vi "IDE_msg_Example.vi"() -> ()   [LabVIEW 2020]
uses:
  Subs/ColorText/Code.xctl
  Subs/Console XCtrl/Console_Xctrl.xctl
  Subs/Server XCtrl/Server.xctl
panel:
  in  "Clean":bool
  in  "PC Save":bool
  in  "PC path":path
  in  "Files":bool
  in  "Server":bool
  in  "Help":bool
  in  "Server":path(xcontrol)=path "/Users/crogers/GitHub/Summer2020/LabVIEWCode/Servers/Jens.vi"
  out "REPL":string(xcontrol)="\nTraceback (most recent call last):\n  File \"<stdin>\", line 1\nSyntaxError: invalid syntax\n>>> print(reply1)\nUnauthorized\n>>> import hub,utime, ujson\n>>> class request:\n...     def __init__(self):\n...         self.ser = hub.USB_VCP()\n...         self.mbegin=b'msg_start\\n'\n...         self.mend=b'\\nmsg_end\\n'\n...         self.rbegin = b'reply_start '\n...         self.rend = b' reply_end'\n...     def comm(self,payload):\n...         s =  b' '\n...         self.ser.write(self.mbegin + payload + self.mend)\n...         utime.sleep(0.01)\n...         while not(self.rend in s):\n...             try:\n...                 s = s + self.ser.readline()\n...             except:\n...                 utime.sleep(0.1)\n...         start = len(self.rbegin)+s.find(self.rbegin)\n...         end = s.find(self.rend)\n...         reply = s[start:end]\n...         return reply.decode()\n...     def put(self, headers, url, data):\n...         request= {\"method\": \"put\",\"headers\": ujson.dumps(headers) ,\"url\": url,\"data\": ujson.dumps(data) }\n...         reply=self.comm(ujson.dumps(request))\n...         utime.sleep(01)\n...         return(reply)\n...     def post(self, headers, url, data):\n...         request= {\"method\": \"post\",\"headers\": ujson.dumps(headers) ,\"url\": url,\"data\": ujson.dumps(data) }\n...         reply=self.comm(ujson.dumps(request))\n...         utime.sleep(01)\n...         return(reply)\n...     def get(self, headers , url):\n...         data = ''\n...         request= {\"method\": \"get\",\"headers\": ujson.dumps(headers) ,\"url\": url,\"data\": ujson.dumps(data)}\n...         reply=self.comm(ujson.dumps(request))\n...         utime.sleep(01)\n...         return(reply)\n... \n>>> test=request()\n>>> SL_Appkey= \"bvd8X9LweQY9o2eP1NYL-p8mLL9wMAk6YYOnYSiIo0\"\n>>> Headers={\"Accept\":\"application/json\",\"x-ni-api-key\": SL_Appkey }\n>>> Url=\"https://api.systemlinkcloud.com/nitag/v2/tags/test1/values/current\"\n>>> Data={\"value\":{\"type\":\"STRING\",\"value\":\"lol\"}}\n>>> reply1=test.get(headers=Headers, url=Url)\nmsg_start\n{\"data\": \"\\\"\\\"\", \"headers\": \"{\\\"x-ni-api-key\\\": \\\"bvd8X9LweQY9o2eP1NYL-p8mLL9wMAk6YYOnYSiIo0\\\", \\\"Accept\\\": \\\"application/json\\\"}\", \"method\": \"get\", \"url\": \"https://api.systemlinkcloud.com/nitag/v2/tags/test1/values/current\"}\nmsg_end\n>>> reply_start Unauthorized reply_endreply_start Unauthorized reply_endreply_start Unauthorized reply_endreply_start Unauthorized reply_endreply_start Unauthorized reply_end\nTraceback (most recent call last):\n  File \"<stdin>\", line 1\nSyntaxError: invalid syntax\n>>> print('hi there')\nhi there\n>>> print(reply1)\nUnauthorized\n>>> "
  in  "Clear":bool
  in  "Save":bool
  in  "Stop":bool
  in  "Run":bool
  in  "Name":string="code.py"
  in  "Code":string(xcontrol)="import hub,utime, ujson\n\nclass request:\n    def __init__(self):\n        self.ser = hub.USB_VCP()\n        self.mbegin=b'msg_start\\n'\n        self.mend=b'\\nmsg_end\\n'\n        self.rbegin = b'reply_start '\n        self.rend = b' reply_end'\n        \n    def comm(self,payload):\n        s =  b' '\n        self.ser.write(self.mbegin + payload + self.mend)\n        utime.sleep(0.01)\n        while not(self.rend in s):\n            try:\n                s = s + self.ser.readline()\n                # print(s)\n            except:\n                utime.sleep(0.1)\n        start = len(self.rbegin)+s.find(self.rbegin)\n        end = s.find(self.rend)\n        reply = s[start:end]\n        return reply.decode()\n        \n    def put(self, headers, url, data):\n        request= {\"method\": \"put\",\"headers\": ujson.dumps(headers) ,\"url\": url,\"data\": ujson.dumps(data) }\n        reply=self.comm(ujson.dumps(request))\n        utime.sleep(01)\n        return(reply)\n        \n    def post(self, headers, url, data):\n        request= {\"method\": \"post\",\"headers\": ujson.dumps(headers) ,\"url\": url,\"data\": ujson.dumps(data) }\n        reply=self.comm(ujson.dumps(request))\n        utime.sleep(01)\n        return(reply)\n        \n    def get(self, headers , url):\n        data = ''\n        request= {\"method\": \"get\",\"headers\": ujson.dumps(headers) ,\"url\": url,\"data\": ujson.dumps(data)}\n        reply=self.comm(ujson.dumps(request))\n        utime.sleep(01)\n        return(reply)\n        \n        \ntest=request()\nSL_Appkey= \"XXX\"\nHeaders={\"Accept\":\"application/json\",\"x-ni-api-key\": SL_Appkey }\nUrl=\"https://api.systemlinkcloud.com/nitag/v2/tags/test1/values/current\"\n\nData={\"value\":{\"type\":\"STRING\",\"value\":\"lol\"}}\n# reply= test.put(headers= Headers , url = Url, data= Data )\n\n\nreply1=test.get(headers=Headers, url=Url)\n\nprint('hi there')\nprint(reply1)\n\n\n"
  # "¨Processor"
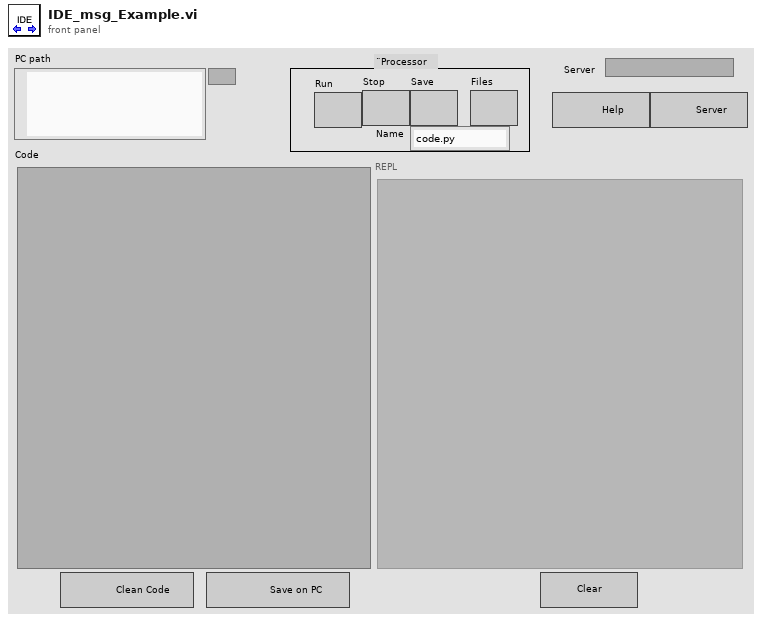
[diagram p1: front panel]
types:
  T1 = cluster{"Quote":u32, "Comment":u32, "Python":u32, "Text":u32, "Triple Quote":u32, "function":u32, "Line numbers":u32, "REPL Err":u32, "REPL Text":u32, "Text Bkgd":u32, "REPL Bkgd":u32}
  T2 = enum8{"Enabled", "Disabled", "Disabled and Grayed Out"}
  T3 = typedef "eventvkey.ctl" = enum16{"ASCII", "Enter", "Return", "Shift", "Ctrl", "Alt", "Cmd", "Opt", "Caps", "NumLock", "Clear", "Break", "Up", "Down", "Left", "Right", "Insert", "Delete", "Home", "End", "PageUp", "PageDown", "Escape", "Help", "Pause", "ScrollLock", "F1", "F2", "F3", "F4", "F5", "F6", "F7", "F8", "F9", "F10", "F11", "F12", "F13", "F14", "F15", "F16", "F17", "F18", "F19", "F20", "F21", "F22", "F23", "F24", "Play", "VolumeUp", "VolumeDown", "Mute", "Two Byte Char"}
  T4 = cluster{"Shift":bool, "Ctrl":bool, "Alt":bool, "Cmd":bool, "Opt":bool}
  T5 = cluster{"Char":i16, "VKey":T3, "PlatMods":cluster{"Shift":bool, "Ctrl":bool, "Alt":bool, "Cmd":bool, "Opt":bool}}
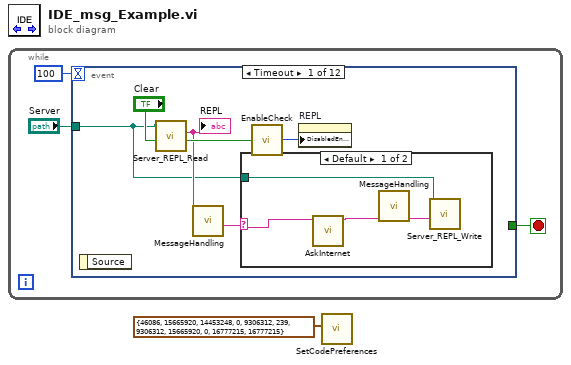
[diagram p0: block diagram]
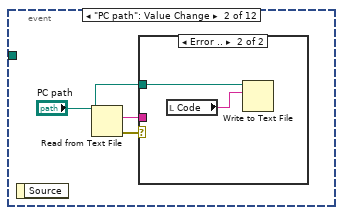
[diagram p3: hidden frame]
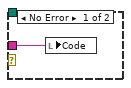
[diagram p4: hidden frame]
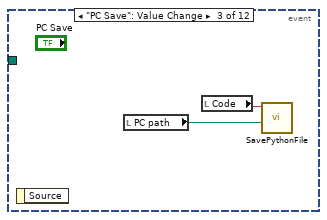
[diagram p5: hidden frame]
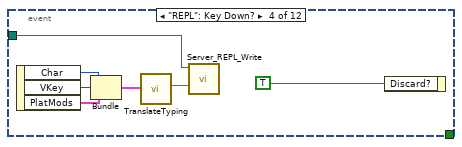
[diagram p6: hidden frame]
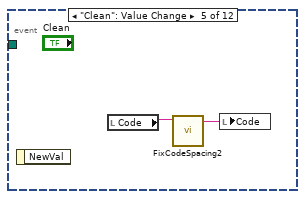
[diagram p7: hidden frame]
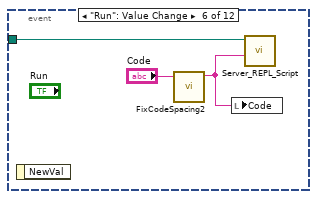
[diagram p8: hidden frame]
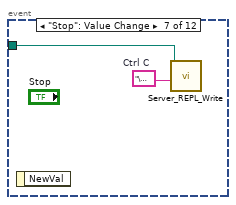
[diagram p9: hidden frame]
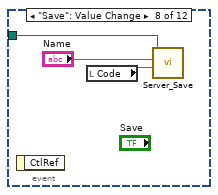
[diagram p10: hidden frame]
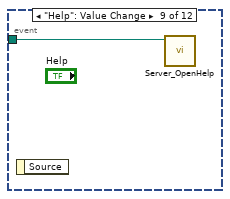
[diagram p11: hidden frame]
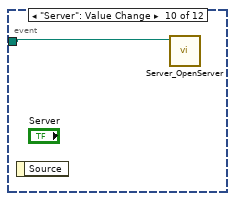
[diagram p12: hidden frame]
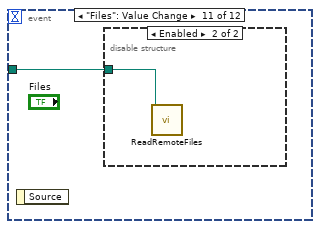
[diagram p13: hidden frame]
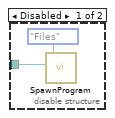
[diagram p14: hidden frame]
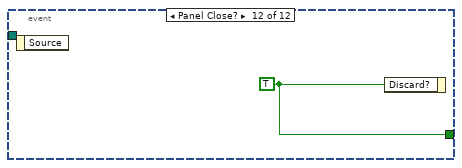
[diagram p15: hidden frame]
diagram:
  n1 = while {
    stop <- w3 stop-if-true
    n2 = event shown="[0] Timeout" {
      selector: _ -> [_ _ _ _ _ _ _ _ _ _ _ _]
      dyn-events: _ -> [_ _ _ _ _ _ _ _ _ _ _ _]
      timeout: 100 -> [_ _ _ _ _ _ _ _ _ _ _ _]
      tunnel: [_ _ _ _ _ _ _ _ _ _ _ w46] -> w3
      tunnel: "Server" -> [w5 _ _ w23 _ w33 w35 w37 w40 w41 w42 _]
      event Timeout {
        n3 = event-data() -> ()  [unwired: 1 in, 1 out]
        n4 = call "Server_REPL_Read.vi"("Clear"="Clear", "Server"=w5) -> ("Running?"=w9:bool, "REPL"=w7:string)  [unwired: 7 in, 1 out]
        "REPL" <- w7
        n5 = call "MessageHandling.vi"("REPL"=w7) -> ("New Message"=w6:string)  [unwired: 7 in, 3 out]
        n6 = case shown="Default" w6 {
          selector: w6 -> [w12 _]
          tunnel: w5 -> [w14 _]
          frame Default {
            n7 = call "AskInternet.vi"("Message Received"=w12) -> ("body"=w11:string)  [unwired: 10 in]
            n8 = call "MessageHandling.vi"("Reply"=w11) -> ("New Reply"=w13:string)  [unwired: 7 in, 3 out]
            n9 = call "Server_REPL_Write.vi"("Code"=w13, "Server"=w14) -> ()  [unwired: 9 in, 1 out]
          }
          frame "" {
          }
        }
        n10 = call "EnableCheck.vi"("Enable?"=w9) -> ("Enum"=w10:T2)
        n11 = property on="REPL" class="Console_Xctrl (strict)"("DisabledEnum"=w10) -> ()  [unwired: 2 in, 2 out]
      }
      event "PC path": Value Change {
        n12 = event-data() -> ()  [unwired: 1 in, 1 out]
        n13 = Read from Text File(file (use dialog)="PC path") -> (text=w16:string, error out=w17:errorcluster)  [unwired: 3 in, 2 out]
        n14 = case shown="Error .." w17 {
          tunnel: w16 -> [w18 _]
          tunnel: "PC path" -> [_ w20]
          frame No Error {
            n15 = local write "Code"(w18) -> ()
          }
          frame Error {
            n16 = local read "Code"() -> (w19:string)
            n17 = Write to Text File(file (use dialog)=w20, text=w19) -> ()  [unwired: 2 in, 3 out]
          }
        }
      }
      event "PC Save": Value Change {
        n18 = event-data() -> ()  [unwired: 1 in, 1 out]
        n19 = local read "PC path"() -> (w21:path)
        n20 = local read "Code"() -> (w22:string)
        n21 = call "SavePythonFile.vi"("path"=w21, "Code"=w22) -> ()  [unwired: 10 in]
      }
      event "REPL": Key Down? {
        n22 = event-data() -> ("Char"=w28:i16, "VKey"=w27:T3, "PlatMods"=w25:T4)  [unwired: 1 in]
        n23 = Bundle("Char"=w28, "VKey"=w27, "PlatMods"=w25) -> (w29:T5)  [unwired: 1 in]
        n24 = call "TranslateTyping.vi"("Cluster"=w29) -> ("key"=w24:string)  [unwired: 10 in]
        n25 = call "Server_REPL_Write.vi"("Code"=w24, "Server"=w23) -> ()  [unwired: 9 in, 1 out]
        n26 = event-data("Discard?"=TRUE) -> ()  [unwired: 1 in, 1 out]
      }
      event "Clean": Value Change {
        n27 = event-data() -> ()  [unwired: 1 in, 1 out]
        n28 = local read "Code"() -> (w30:string)
        n29 = call "FixCodeSpacing2.vi"("Code"=w30) -> ("Cleaned"=w31:string)  [unwired: 10 in]
        n30 = local write "Code"(w31) -> ()
      }
      event "Run": Value Change {
        n31 = event-data() -> ()  [unwired: 1 in, 1 out]
        n32 = call "FixCodeSpacing2.vi"("Code"="Code") -> ("Cleaned"=w32:string)  [unwired: 10 in]
        n33 = local write "Code"(w32) -> ()
        n34 = call "Server_REPL_Script.vi"("Code"=w32, "Server"=w33) -> ()  [unwired: 9 in, 1 out]
      }
      event "Stop": Value Change {
        w36 = "\u0003"  # Ctrl C
        n35 = event-data() -> ()  [unwired: 1 in, 1 out]
        n36 = call "Server_REPL_Write.vi"("Code"=w36, "Server"=w35) -> ()  [unwired: 9 in, 1 out]
      }
      event "Save": Value Change {
        n37 = event-data() -> ()  [unwired: 1 in, 1 out]
        n38 = local read "Code"() -> (w39:string)
        n39 = call "Server_Save.vi"("Code"=w39, "Name"="Name", "Server"=w37) -> ()  [unwired: 8 in, 1 out]
      }
      event "Help": Value Change {
        n40 = event-data() -> ()  [unwired: 1 in, 1 out]
        n41 = call "Server_OpenHelp.vi"("Server"=w40) -> ()  [unwired: 10 in, 1 out]
      }
      event "Server": Value Change {
        n42 = event-data() -> ()  [unwired: 1 in, 1 out]
        n43 = call "Server_OpenServer.vi"("Server"=w41) -> ()  [unwired: 10 in, 1 out]
      }
      event "Files": Value Change {
        n44 = event-data() -> ()  [unwired: 1 in, 1 out]
        n45 = disable-structure shown="Enabled" {
          disable-tunnel: w42 -> [w43 w45]
          frame Disabled {
            n46 = call "SpawnProgram.vi"("Server"=w43, "Dialog"=enum16{"Help", "Files"}."Files") -> ()  [unwired: 10 in]
          }
          frame Enabled {
            n47 = call "ReadRemoteFiles.vi"("Server"=w45) -> ()  [unwired: 11 in]
          }
        }
      }
      event Panel Close? {
        w46 = TRUE ("Discard?")
        n48 = event-data() -> ()  [unwired: 1 in, 1 out]
        n49 = event-data("Discard?"=w46) -> ()  [unwired: 1 in, 1 out]
      }
    }
  }
  n50 = call "SetCodePreferences.vi"("Color choices"=T1 {"Quote"=46086, "Comment"=15665920, "Python"=14453248, "Text"=0, "Triple Quote"=9306312, "function"=239, "Line numbers"=9306312, "REPL Err"=15665920, "REPL Text"=0, "Text Bkgd"=16777215, "REPL Bkgd"=16777215}) -> ()  [unwired: 11 in]
